vi "SQL_Template_insertbyname.vi"(8 "创建时间":string, 10 "创建人":string, 11 "tempName":string) -> (3 "error out":errorcluster)   [LabVIEW 2014]
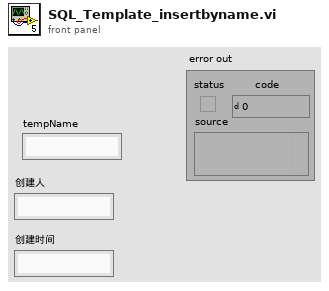
[diagram p1: front panel]
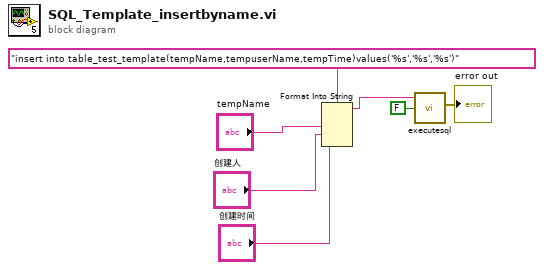
[diagram p0: block diagram]
diagram:
  n1 = Format Into String(format string="insert into table_test_template(tempName,tempuserName,tempTime)values('%s','%s','%s')", "tempName", "创建人", "创建时间") -> (resulting string=w5:string)  [unwired: 2 in, 1 out]
  n2 = call "executesql.vi"("Return Data (T)"=FALSE, "Command Text"=w5) -> ("error out"=→"error out":errorcluster)  [unwired: 5 in, 1 out]
